vi "ReadAddError__slk_mt.vi"(8 "error in (no error)":errorcluster, 11 "refnum in":T1) -> (0 "error out":errorcluster, 2 "add error configure":T2, 3 "refnum out":T1)   [LabVIEW 2012, in "Lazyboots Menu Tool.lvlib"]
doc: "Gets configure datum of Add Error.\n\n<b>[Add Error]</b>\nFrame Width = \"20\"\nAlign to Grid = \"TRUE\"\nFP Grid Size = \"10\"\nWire to Connector = \"TRUE\"\nConnector Pattern = \"4815\"\nControl Style = \"Classic Style\"\nError Style = \"2 Columns Style\""
uses:
  Library/Lazyboots Menu Tool.lvlib
  <vilib>/Utility/config.llb/NI_LVConfig.lvlib
  <vilib>/Utility/config.llb/Read Key (Boolean).vi
  TypeDef/TypeDef_AddErrorConfigure__slk_mt.ctl
  <vilib>/Utility/config.llb/Read Key (U32).vi
  <vilib>/Utility/config.llb/Read Key (String).vi
  <vilib>/Utility/config.llb/Config Data RefNum.ctl
panel:
  # "ReadAddError__slk_mt.vi\nGets configure datum of Add Error.\n\nNOTICE -- YOU MUST LEAVE THIS NOTICE IN PLACE.\n\nCopyright (c) 2011, LIANG LIU Shawn.Liu.cn@gmail.com\nAll rights reserved.\n\nRedistribution and use in source and binary forms, with or without modification, are permitted provided that the following conditions are met:\n-Redistributions of source code must retain the above copyright notice, this list of conditions and the following disclaimer.\n-Redistributions in binary form must reproduce the above copyright notice, this list of conditions and the following disclaimer in the documentation and/or other materials provided with the distribution.\n-Neither the name of the eLp nor the names of its contributors may be used to endorse or promote products derived from this software without specific prior written permission.\n\nTHIS SOFTWARE IS PROVIDED BY THE COPYRIGHT HOLDERS AND CONTRIBUTORS \"AS IS\" AND ANY EXPRESS OR IMPLIED WARRANTIES, INCLUDING, BUT NOT LIMITED TO, THE IMPLIED WARRANTIES OF MERCHANTABILITY AND FITNESS FOR A PARTICULAR PURPOSE ARE DISCLAIMED. IN NO EVENT SHALL THE COPYRIGHT HOLDER OR CONTRIBUTORS BE LIABLE FOR ANY DIRECT, INDIRECT, INCIDENTAL, SPECIAL, EXEMPLARY, OR CONSEQUENTIAL DAMAGES (INCLUDING, BUT NOT LIMITED TO, PROCUREMENT OF SUBSTITUTE GOODS OR SERVICES; LOSS OF USE, DATA, OR PROFITS; OR BUSINESS INTERRUPTION) HOWEVER CAUSED AND ON ANY THEORY OF LIABILITY, WHETHER IN CONTRACT, STRICT LIABILITY, OR TORT (INCLUDING NEGLIGENCE OR OTHERWISE) ARISING IN ANY WAY OUT OF THE USE OF THIS SOFTWARE, EVEN IF ADVISED OF THE POSSIBILITY OF SUCH DAMAGE."
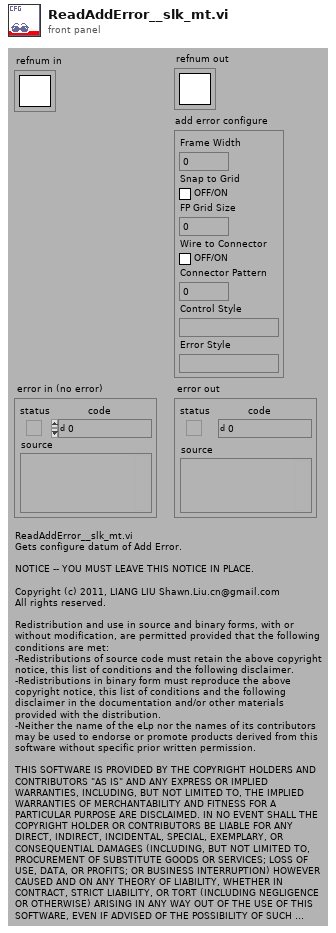
[diagram p1: front panel]
types:
  T1 = typedef "NI_LVConfig.lvlib/Config Data RefNum.ctl" = refnum<k1>
  T2 = typedef "Lazyboots Menu Tool.lvlib/TypeDef_AddErrorConfigure__slk_mt.ctl" = cluster{"Frame Width":u32, "Snap to Grid":bool, "FP Grid Size":u32, "Wire to Connector":bool, "Connector Pattern":u32, "Control Style":string, "Error Style":string}
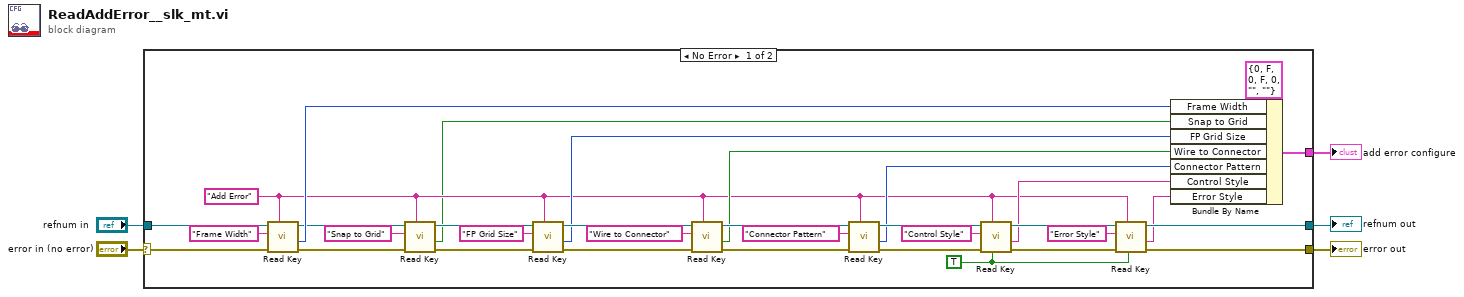
[diagram p0: block diagram]
diagram:
  n1 = case shown="No Error" "error in (no error)" {
    selector: "error in (no error)" -> [w34 w41]
    tunnel: [w35 _] -> w5
    tunnel: [w15 w41] -> w4
    tunnel: "refnum in" -> [w33 w40]
    tunnel: [w22 w40] -> w1
    frame No Error {
      w14 = TRUE ("read raw string? (F)")
      w10 = "Add Error" ("section")
      n2 = call-poly <vilib>:"Read Key.vi"("section"=w10, "error in (no error)"=w34, "key"="Frame Width", "refnum"=w33) -> ("error out"=w9:errorcluster, "value"=w36:u32, "refnum out"=w12:T1)  [unwired: 4 in, 1 out]
      n3 = call-poly <vilib>:"Read Key.vi"("section"=w10, "error in (no error)"=w9, "key"="Snap to Grid", "refnum"=w12) -> ("error out"=w8:errorcluster, "value"=w6:bool, "refnum out"=w11:T1)  [unwired: 4 in, 1 out]
      n4 = call-poly <vilib>:"Read Key.vi"("section"=w10, "error in (no error)"=w8, "key"="FP Grid Size", "refnum"=w11) -> ("error out"=w29:errorcluster, "value"=w13:u32, "refnum out"=w32:T1)  [unwired: 4 in, 1 out]
      n5 = call-poly <vilib>:"Read Key.vi"("section"=w10, "error in (no error)"=w29, "key"="Wire to Connector", "refnum"=w32) -> ("error out"=w26:errorcluster, "value"=w28:bool, "refnum out"=w31:T1)  [unwired: 4 in, 1 out]
      n6 = call-poly <vilib>:"Read Key.vi"("section"=w10, "error in (no error)"=w26, "key"="Connector Pattern", "refnum"=w31) -> ("error out"=w21:errorcluster, "value"=w24:u32, "refnum out"=w27:T1)  [unwired: 4 in, 1 out]
      n7 = call-poly <vilib>:"Read Key.vi"("read raw string? (F)"=w14, "section"=w10, "error in (no error)"=w21, "key"="Control Style", "refnum"=w27) -> ("error out"=w18:errorcluster, "value"=w17:string, "refnum out"=w23:T1)  [unwired: 3 in, 1 out]
      n8 = call-poly <vilib>:"Read Key.vi"("read raw string? (F)"=w14, "section"=w10, "error in (no error)"=w18, "key"="Error Style", "refnum"=w23) -> ("error out"=w15:errorcluster, "value"=w16:string, "refnum out"=w22:T1)  [unwired: 3 in, 1 out]
      n9 = Bundle By Name(cluster=T2 {"Frame Width"=0, "Snap to Grid"=FALSE, "FP Grid Size"=0, "Wire to Connector"=FALSE, "Connector Pattern"=0, "Control Style"="", "Error Style"=""} ("Add Error Configure"), "Frame Width"=w36, "Snap to Grid"=w6, "FP Grid Size"=w13, "Wire to Connector"=w28, "Connector Pattern"=w24, "Control Style"=w17, "Error Style"=w16) -> (w35:T2)
    }
    frame Error {
    }
  }
  "add error configure" <- w5
  "error out" <- w4
  "refnum out" <- w1
